vi "Scaling data (from 0.5 to 0.95).vi"(0 "Input data":sgl[](array[numeric]) format="%.2f") -> (1 "Offset up":sgl format="%.2f", 2 "Offset down":sgl format="%.2f", 3 "Scaled data":sgl[](array[numeric]) format="%.2f")   [LabVIEW 2010]
doc: "This VI scales the data from any range (also negative) into linear range in such a way that minimum input = 0.05 and maximum input = 0.95."
panel:
  out "back scaled data":sgl[](array[numeric]) format="%.2f"
  out "no low offset":sgl[](array[numeric]) format="%.2f"
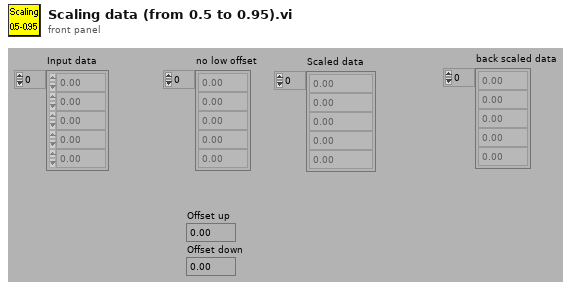
[diagram p1: front panel]
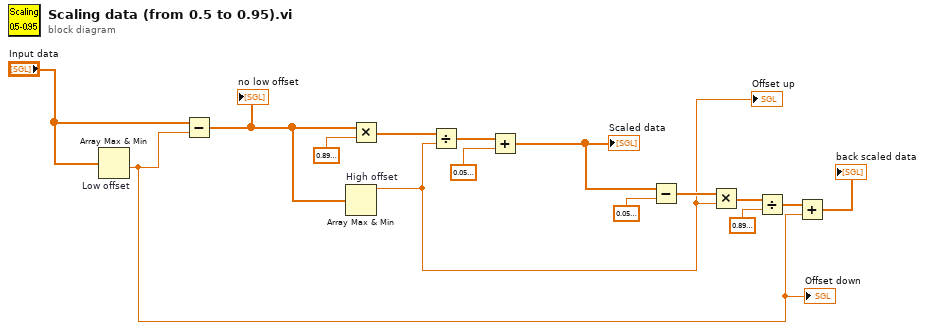
[diagram p0: block diagram]
diagram:
  n1 = Array Max & Min "Low offset"(array="Input data") -> (min value=w4:sgl)  [unwired: 3 out]
  "Offset down" <- w4
  n2 = Subtract(x="Input data", y=w4) -> (x-y=w13:sgl[])
  "no low offset" <- w13
  n3 = Array Max & Min "High offset"(array=w13) -> (max value=w8:sgl)  [unwired: 3 out]
  "Offset up" <- w8
  n4 = Multiply(x=w13, y=sgl 0.9 ("x")) -> (x*y=w14:sgl[])
  n5 = Divide(x=w14, y=w8) -> (x/y=w12:sgl[])
  n6 = Add(x=w12, y=sgl 0.05) -> (x+y=w1:sgl[])
  "Scaled data" <- w1
  n7 = Subtract(x=w1, y=sgl 0.05) -> (x-y=w9:sgl[])
  n8 = Multiply(x=w9, y=w8) -> (x*y=w7:sgl[])
  n9 = Divide(x=w7, y=sgl 0.9 ("x")) -> (x/y=w5:sgl[])
  n10 = Add(x=w5, y=w4) -> (x+y=→"back scaled data":sgl[])
